vi "Anzeige.vi"(0 "AIs":dbl[](array[numeric]), 1 "Zykluslängen [s]":dbl[](array[numeric]), 2 "Cluster1":cluster{dbl[], dbl[], dbl[], dbl[]}, 3 "veränderte Methode benutzen":bool, 4 "Big Ben, Methodenzeit, Zykluszeit0, Zykluszeit1, Zykluszeit2A, Zykluszeit2B":dbl[](array[numeric]), 5 "Zyklusnummern 0, 1, 2A, 2B":i32[](array[numeric]), 6 "Cluster2":cluster{dbl[], dbl[], dbl[], dbl[]}, 7 "AnzeigeEinstellungen":T1, 8 "Tafel putzen2":bool, 9 "Tafel putzen1":bool, 11 "MWHorst":dbl[](array[numeric]), 12 "Traps/Machs":dbl[](array[numeric]), 13 "dargestellte Größe 1":i32(ring)=1 items=["T-MainCol3", "T-Trap1", "T-Trap2", "T-Stirling", "T-PreCol1", "T-PreCol2", "T-MainCol1", "T-MainCol2", "T-T-Line2", "T-MI1", "T-MI2", "T-MI3", "T-MI4", "T-MI5", "T-MI6", "F-MFM1", "T-MainCol4", "T-BHorst1", "T-BHorst2", "T-BHorst3", "T-BHorst4", "T-Oven1", "T-Oven2", "T-T-Line1", "F-MFM2", "P-Me-HP", "P-Me-LP", "P-Vac", "Ref-Turbo", "I-MS-AC", "I-Trap1", "I-Trap2", "Mod2/AI0", "Mod2/AI1", "Mod2/AI2", "Mod2/AI3", "Mod2/AI4", "Mod2/AI5", "Mod2/AI6", "Mod2/AI7", "Mod2/AI8", "Mod2/AI9", "Mod2/AI10", "Mod2/AI11", "Mod2/AI12", "Mod2/AI13", "Mod2/AI14", "Mod2/AI15", "Mod2/AI16", "Mod2/AI17", "Mod2/AI18", "Mod2/AI19", "Mod2/AI20", "Mod2/AI21", "Mod2/AI22", "Mod2/AI23", "Mod2/AI24", "Mod2/AI25", "Mod2/AI26", "Mod2/AI27", "Mod2/AI28", "Mod2/AI29", "Mod2/AI30", "Mod2/AI31", "Mod3/AI0", "Mod3/AI1", "Mod3/AI2", "Mod3/AI3", "Mod3/AI4", "Mod3/AI5", "Mod3/AI6", "Mod3/AI7", "Mod3/AI8", "Mod3/AI9", "Mod3/AI10", "Mod3/AI11", "Mod3/AI12", "Mod3/AI13", "Mod3/AI14", "Mod3/AI15", "Mod3/AI16", "Mod3/AI17", "Mod3/AI18", "Mod3/AI19", "Mod3/AI20", "Mod3/AI21", "Mod3/AI22", "Mod3/AI23", "Mod3/AI24", "Mod3/AI25", "Mod3/AI26", "Mod3/AI27", "Mod3/AI28", "Mod3/AI29", "Mod3/AI30", "Mod3/AI31", "U_Widr.Trap1 [V]", "Temp.Trap1 [°C]", "U_Widr.Trap2 [V]", "Temp.Trap2 [°C]", "Temp.Mach1 [°C]", "Temp.Mach2 [°C]", "MFC1B", "PressContr1A", "PressContr1B", "PressContr1C", "MFC1A", "PressContr1D", "MFC1A Integriert"], 14 "Zeitachse1":i32(ring)=1 items=["Zykluszeit [s] Mod0", "Zykluszeit [s] Mod1", "Zykluszeit [s] Mod2A", "Zykluszeit [s] Mod2B"], 15 "Zeitachse2":i32(ring)=1 items=["Zykluszeit [s] Mod0", "Zykluszeit [s] Mod1", "Zykluszeit [s] Mod2A", "Zykluszeit [s] Mod2B"], 16 "dargestellte Größe 2":i32(ring)=1 items=["T-MainCol3", "T-Trap1", "T-Trap2", "T-Stirling", "T-PreCol1", "T-PreCol2", "T-MainCol1", "T-MainCol2", "T-T-Line2", "T-MI1", "T-MI2", "T-MI3", "T-MI4", "T-MI5", "T-MI6", "F-MFM1", "T-MainCol4", "T-BHorst1", "T-BHorst2", "T-BHorst3", "T-BHorst4", "T-Oven1", "T-Oven2", "T-T-Line1", "F-MFM2", "P-Me-HP", "P-Me-LP", "P-Vac", "Ref-Turbo", "I-MS-AC", "I-Trap1", "I-Trap2", "Mod2/AI0", "Mod2/AI1", "Mod2/AI2", "Mod2/AI3", "Mod2/AI4", "Mod2/AI5", "Mod2/AI6", "Mod2/AI7", "Mod2/AI8", "Mod2/AI9", "Mod2/AI10", "Mod2/AI11", "Mod2/AI12", "Mod2/AI13", "Mod2/AI14", "Mod2/AI15", "Mod2/AI16", "Mod2/AI17", "Mod2/AI18", "Mod2/AI19", "Mod2/AI20", "Mod2/AI21", "Mod2/AI22", "Mod2/AI23", "Mod2/AI24", "Mod2/AI25", "Mod2/AI26", "Mod2/AI27", "Mod2/AI28", "Mod2/AI29", "Mod2/AI30", "Mod2/AI31", "Mod3/AI0", "Mod3/AI1", "Mod3/AI2", "Mod3/AI3", "Mod3/AI4", "Mod3/AI5", "Mod3/AI6", "Mod3/AI7", "Mod3/AI8", "Mod3/AI9", "Mod3/AI10", "Mod3/AI11", "Mod3/AI12", "Mod3/AI13", "Mod3/AI14", "Mod3/AI15", "Mod3/AI16", "Mod3/AI17", "Mod3/AI18", "Mod3/AI19", "Mod3/AI20", "Mod3/AI21", "Mod3/AI22", "Mod3/AI23", "Mod3/AI24", "Mod3/AI25", "Mod3/AI26", "Mod3/AI27", "Mod3/AI28", "Mod3/AI29", "Mod3/AI30", "Mod3/AI31", "U_Widr.Trap1 [V]", "Temp.Trap1 [°C]", "U_Widr.Trap2 [V]", "Temp.Trap2 [°C]", "Temp.Mach1 [°C]", "Temp.Mach2 [°C]", "MFC1B", "PressContr1A", "PressContr1B", "PressContr1C", "MFC1A", "PressContr1D", "MFC1A Integriert"], 17 "Methodenwechsel?":bool) -> (19 "Anzeige2":cluster{dbl[], dbl[]}(graph), 20 "Cluster1":cluster{dbl[], dbl[], dbl[], dbl[]}, 21 "x1Inkr":dbl, 22 "Cluster2":cluster{dbl[], dbl[], dbl[], dbl[]}, 23 "Anzeige1":cluster{dbl[], dbl[]}(graph), 24 "AnzeigeEinstellungen":T1, 25 "x2Max":dbl, 26 "x2Inkr":dbl, 27 "x1Max":dbl)   [LabVIEW 2010]
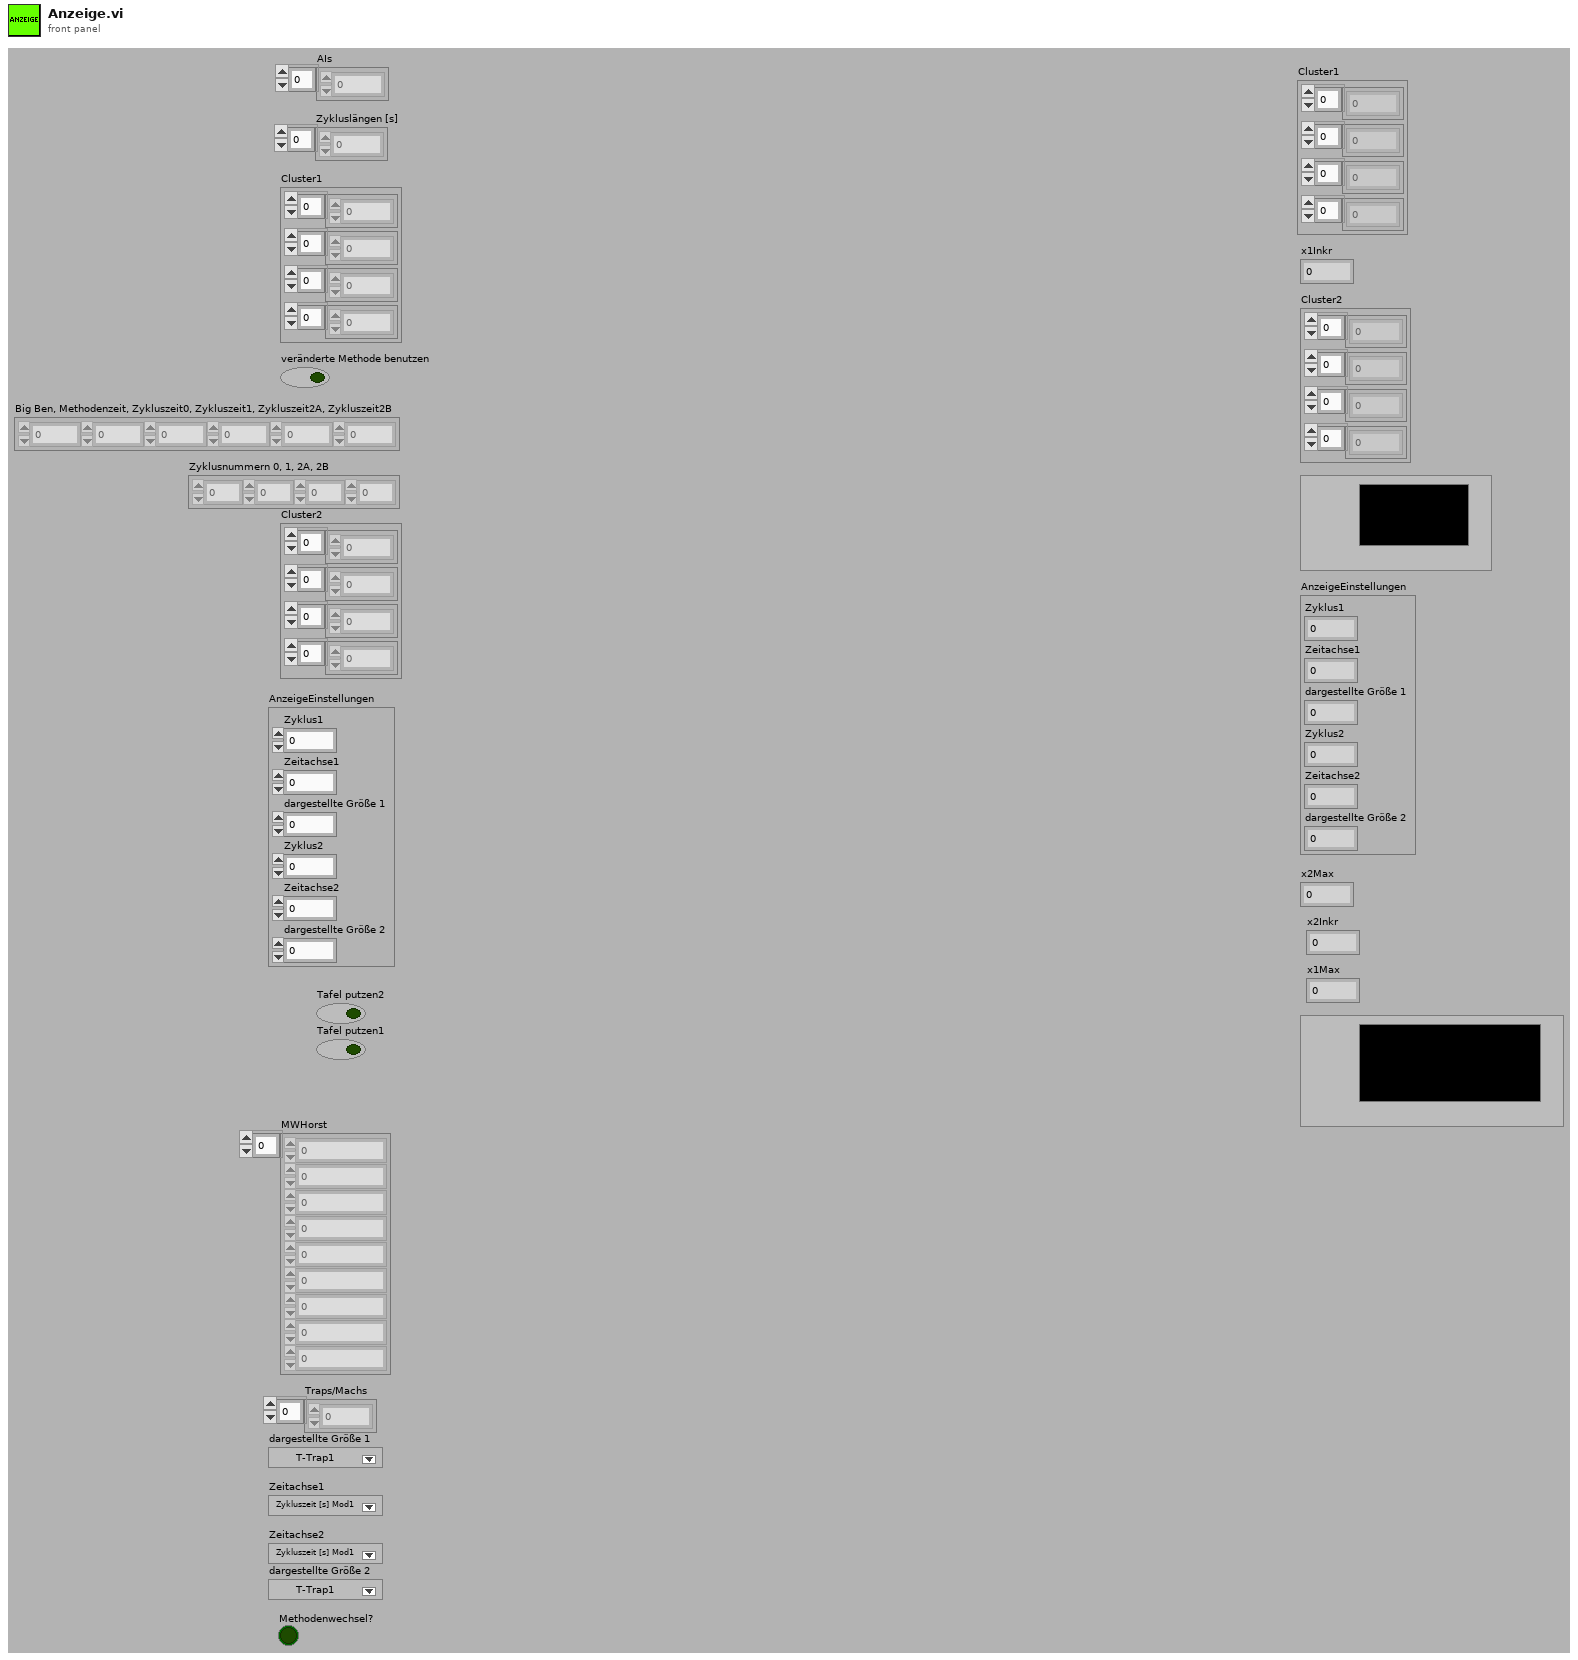
[diagram p1: front panel]
types:
  T1 = cluster{"Zyklus1":i32, "Zeitachse1":i32, "dargestellte Größe 1":i32, "Zyklus2":i32, "Zeitachse2":i32, "dargestellte Größe 2":i32}
  T2 = cluster{i32, "Zeitachse1":i32, "dargestellte Größe 1":i32, i32, "Zeitachse2":i32, "dargestellte Größe 2":i32}
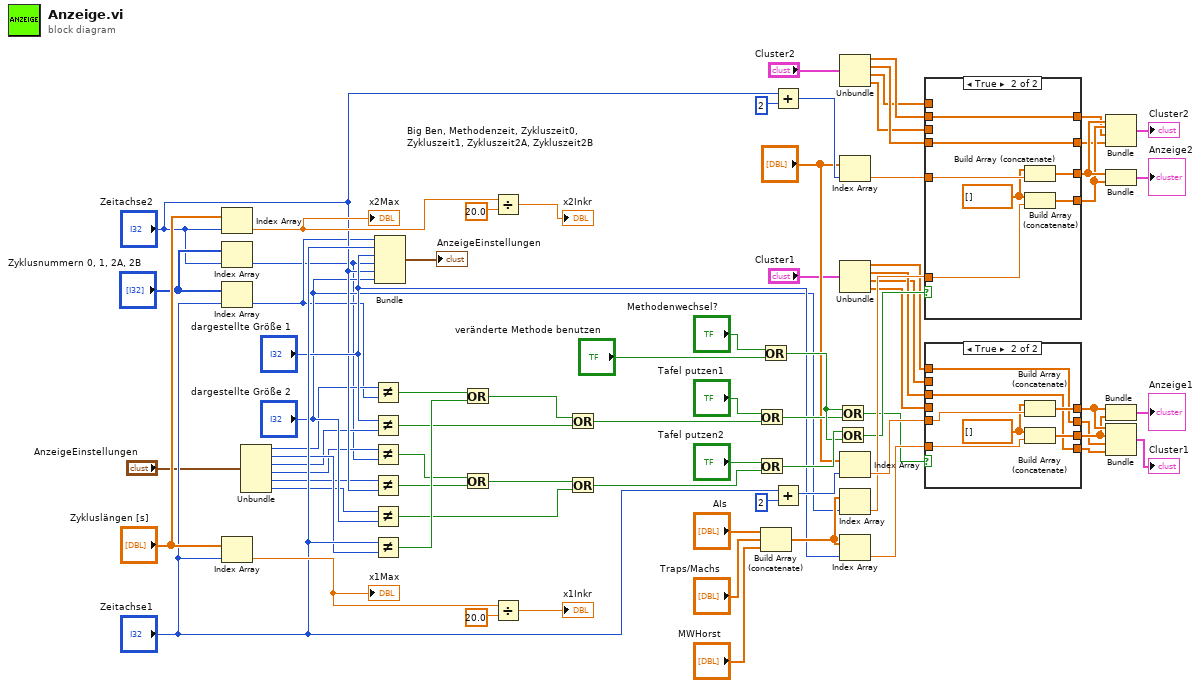
[diagram p0: block diagram]
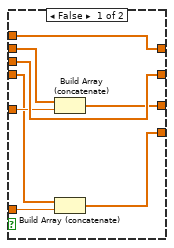
[diagram p2: hidden frame]
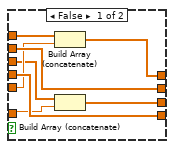
[diagram p3: hidden frame]
diagram:
  n1 = Index Array(array="Zykluslängen [s]", index="Zeitachse2") -> (element=w18:dbl)
  "x2Max" <- w18
  n2 = Index Array(array="Zyklusnummern 0, 1, 2A, 2B", index="Zeitachse2") -> (element=w3:i32)
  n3 = Index Array(array="Zyklusnummern 0, 1, 2A, 2B", index="Zeitachse1") -> (element=w7:i32)
  n4 = Index Array(array="Zykluslängen [s]", index="Zeitachse1") -> (element=w16:dbl)
  "x1Max" <- w16
  n5 = Unbundle("AnzeigeEinstellungen") -> ("Zyklus1"=w8:i32, "Zeitachse1"=w6:i32, "dargestellte Größe 1"=w5:i32, "Zyklus2"=w4:i32, "Zeitachse2"=w2:i32, "dargestellte Größe 2"=w1:i32)
  n6 = Not Equal?(x=w8, y=w7) -> (x != y?=w73:bool)
  n7 = Not Equal?(x="dargestellte Größe 1", y=w5) -> (x != y?=w70:bool)
  n8 = Not Equal?(x=w4, y=w3) -> (x != y?=w65:bool)
  n9 = Not Equal?(x=w2, y="Zeitachse2") -> (x != y?=w64:bool)
  n10 = Not Equal?(x=w1, y="dargestellte Größe 2") -> (x != y?=w62:bool)
  n11 = Not Equal?(x="Zeitachse1", y=w6) -> (x != y?=w71:bool)
  n12 = Bundle(w7, "Zeitachse1"="Zeitachse1", "dargestellte Größe 1"="dargestellte Größe 1", w3, "Zeitachse2"="Zeitachse2", "dargestellte Größe 2"="dargestellte Größe 2") -> (→"AnzeigeEinstellungen":T2)  [unwired: 1 in]
  n13 = Or(x=w73, y=w71) -> (x .or. y?=w72:bool)
  n14 = Or(x=w65, y=w64) -> (x .or. y?=w63:bool)
  n15 = Divide(x=w18, y=20.0) -> (x/y=→"x2Inkr":dbl)
  n16 = Divide(x=w16, y=20.0) -> (x/y=→"x1Inkr":dbl)
  n17 = Or(x=w72, y=w70) -> (x .or. y?=w59:bool)
  n18 = Or(x=w63, y=w62) -> (x .or. y?=w60:bool)
  n19 = Or(x="Tafel putzen1", y=w59) -> (x .or. y?=w48:bool)
  n20 = Or(x="Tafel putzen2", y=w60) -> (x .or. y?=w51:bool)
  n21 = Or(x="Methodenwechsel?", y="veränderte Methode benutzen") -> (x .or. y?=w49:bool)
  n22 = Build Array (concatenate)("AIs", "Traps/Machs", "MWHorst") -> (w68:dbl[])
  n23 = Add(x="Zeitachse2", y=2) -> (x+y=w56:i32)
  n24 = Add(x="Zeitachse1", y=2) -> (x+y=w55:i32)
  n25 = Or(x=w49, y=w48) -> (x .or. y?=w47:bool)
  n26 = Or(x=w51, y=w49) -> (x .or. y?=w50:bool)
  n27 = Unbundle("Cluster2") -> (w46:dbl[], w45:dbl[], w44:dbl[], w43:dbl[])
  n28 = Index Array(array="Big Ben, Methodenzeit, Zykluszeit0, Zykluszeit1, Zykluszeit2A, Zykluszeit2B", index=w56) -> (element=w66:dbl)
  n29 = Unbundle("Cluster1") -> (w37:dbl[], w36:dbl[], w35:dbl[], w34:dbl[])
  n30 = Index Array(array="Big Ben, Methodenzeit, Zykluszeit0, Zykluszeit1, Zykluszeit2A, Zykluszeit2B", index=w55) -> (element=w75:dbl)
  n31 = Index Array(array=w68, index="dargestellte Größe 2") -> (element=w67:dbl)
  n32 = Index Array(array=w68, index="dargestellte Größe 1") -> (element=w74:dbl)
  n33 = case shown="True" w50 {
    tunnel: w46 -> [w82 w86]
    tunnel: [w80 w90] -> w42
    tunnel: [w77 w87] -> w41
    tunnel: w44 -> [w84 _]
    tunnel: [w84 w86] -> w40
    tunnel: w43 -> [w83 _]
    tunnel: [w83 w85] -> w39
    tunnel: w66 -> [w81 w91]
    tunnel: w45 -> [w79 w85]
    tunnel: w67 -> [w78 w88]
    frame False {
      n34 = Build Array (concatenate)(w82, w81) -> (w80:dbl[])
      n35 = Build Array (concatenate)(w79, w78) -> (w77:dbl[])
    }
    frame True {
      w89 = dbl[] []
      n36 = Build Array (concatenate)(w89, w91) -> (w90:dbl[])
      n37 = Build Array (concatenate)(w89, w88) -> (w87:dbl[])
    }
  }
  n38 = case shown="True" w47 {
    tunnel: w37 -> [w97 w101]
    tunnel: [w95 w105] -> w33
    tunnel: [w92 w102] -> w32
    tunnel: w35 -> [w99 _]
    tunnel: [w99 w101] -> w31
    tunnel: w34 -> [w98 _]
    tunnel: [w98 w100] -> w30
    tunnel: w75 -> [w96 w106]
    tunnel: w36 -> [w94 w100]
    tunnel: w74 -> [w93 w103]
    frame False {
      n39 = Build Array (concatenate)(w97, w96) -> (w95:dbl[])
      n40 = Build Array (concatenate)(w94, w93) -> (w92:dbl[])
    }
    frame True {
      w104 = dbl[] []
      n41 = Build Array (concatenate)(w104, w106) -> (w105:dbl[])
      n42 = Build Array (concatenate)(w104, w103) -> (w102:dbl[])
    }
  }
  n43 = Bundle(w42, w41, w40, w39) -> (→"Cluster2":cluster{dbl[], dbl[], dbl[], dbl[]})  [unwired: 1 in]
  n44 = Bundle(w42, w41) -> (→"Anzeige2":cluster{dbl[], dbl[]})  [unwired: 1 in]
  n45 = Bundle(w33, w32) -> (→"Anzeige1":cluster{dbl[], dbl[]})  [unwired: 1 in]
  n46 = Bundle(w33, w32, w31, w30) -> (→"Cluster1":cluster{dbl[], dbl[], dbl[], dbl[]})  [unwired: 1 in]
